vi "simularea_efectelor_grafice.vi"() -> ()   [LabVIEW 2025]
panel:
  out "DESCRIERE EFECT GRAFIC":string
  out "L 32":bool
  out "L 31":bool
  out "L 30":bool
  out "L 29":bool
  out "L 28":bool
  out "L 27":bool
  out "L 26":bool
  out "L 25":bool
  out "L 24":bool
  out "L 23":bool
  out "L 22":bool
  out "L 21":bool
  out "L 20":bool
  out "L 19":bool
  out "L 18":bool
  out "L 17":bool
  out "L 16":bool
  out "L 15":bool
  out "L 14":bool
  out "L 13":bool
  out "L 12":bool
  out "L 11":bool
  out "L 10":bool
  out "L 9":bool
  out "L 8":bool
  out "L 7":bool
  out "L 6":bool
  out "L 5":bool
  out "L 4":bool
  out "L 3":bool
  out "L 2":bool
  out "L 1":bool
  in  "VITEZA EFECT":i32(knob) scale=100.0..2000.0
  in  "SELECTOR-EFECTE GRAFICE":string(combo)
  in  "stop":bool
  # "marire dimensiune text -tastatura setata pe engleza(uk sau us)\n                                          - CTRL + SHIFT + >"
  # "SIMULAREA EFECTELOR GRAFICE CARE POT FI AFISATE LA NIVELUL MATRICEI CU 8x4 LEDURI"
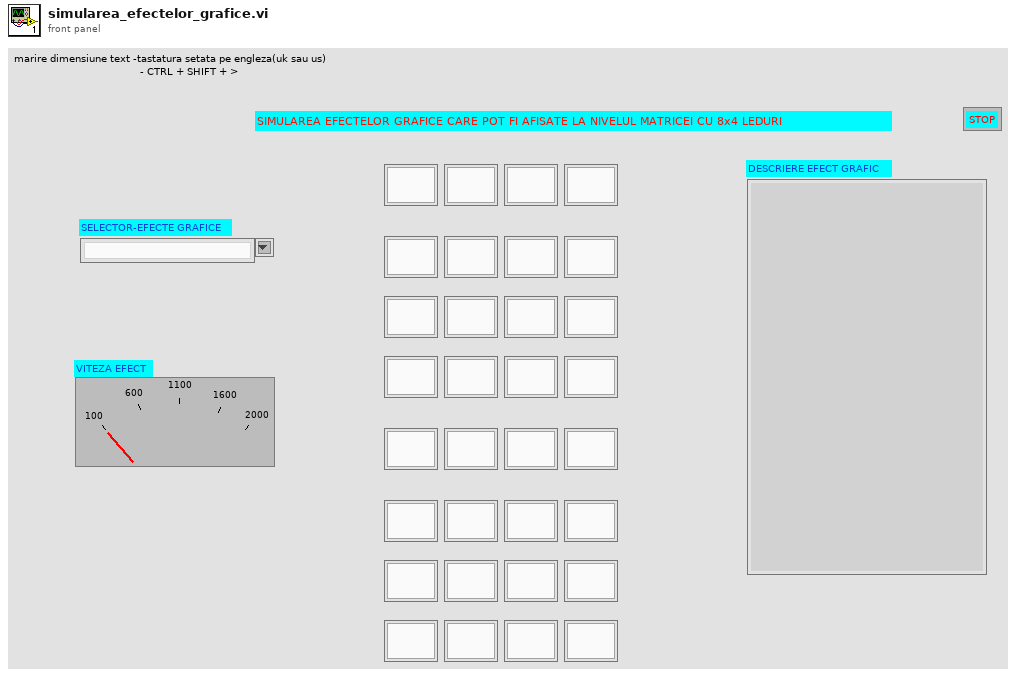
[diagram p1: front panel]
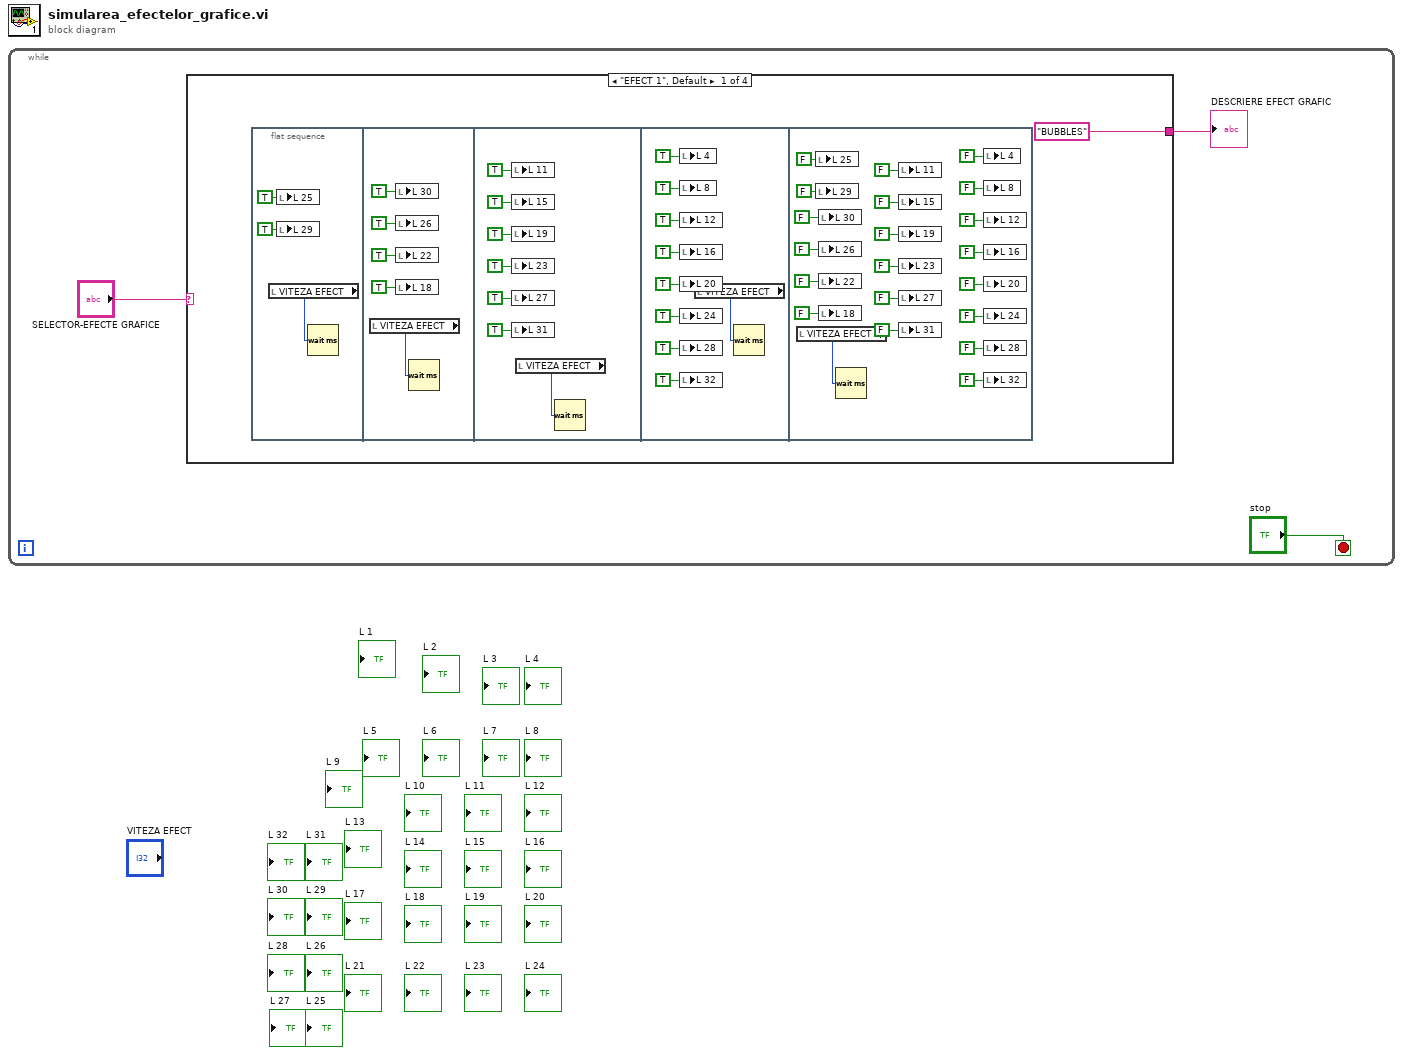
[diagram p0: block diagram]
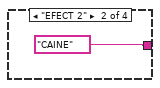
[diagram p2: hidden frame]
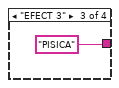
[diagram p3: hidden frame]
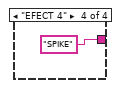
[diagram p4: hidden frame]
diagram:
  n1 = while {
    stop <- "stop" stop-if-true
    n2 = case shown="\"EFECT 1\", Default" "SELECTOR-EFECTE GRAFICE" {
      tunnel: ["BUBBLES" "CAINE" "PISICA" "SPIKE"] -> w1
      frame "EFECT 1", Default {
        n3 = flat-sequence {
          frame #0 {
            n4 = local read "VITEZA EFECT"() -> (w5:i32)
            n5 = local write "L 25"(TRUE ("L 25")) -> ()
            n6 = local write "L 29"(TRUE ("L 29")) -> ()
            n7 = Wait (ms)(milliseconds to wait=w5) -> ()  [unwired: 1 out]
          }
          frame #1 {
            n8 = local read "VITEZA EFECT"() -> (w8:i32)
            n9 = local write "L 30"(TRUE ("L 30")) -> ()
            n10 = local write "L 26"(TRUE ("L 26")) -> ()
            n11 = local write "L 22"(TRUE ("L 22")) -> ()
            n12 = local write "L 18"(TRUE ("L 18")) -> ()
            n13 = Wait (ms)(milliseconds to wait=w8) -> ()  [unwired: 1 out]
          }
          frame #2 {
            n14 = local write "L 11"(TRUE ("L 11")) -> ()
            n15 = local write "L 15"(TRUE ("L 15")) -> ()
            n16 = local write "L 19"(TRUE ("L 19")) -> ()
            n17 = local write "L 23"(TRUE ("L 23")) -> ()
            n18 = local write "L 27"(TRUE ("L 27")) -> ()
            n19 = local write "L 31"(TRUE ("L 31")) -> ()
            n20 = local read "VITEZA EFECT"() -> (w13:i32)
            n21 = Wait (ms)(milliseconds to wait=w13) -> ()  [unwired: 1 out]
          }
          frame #3 {
            n22 = local write "L 4"(TRUE ("L 4")) -> ()
            n23 = local write "L 8"(TRUE ("L 8")) -> ()
            n24 = local write "L 12"(TRUE ("L 12")) -> ()
            n25 = local write "L 16"(TRUE ("L 16")) -> ()
            n26 = local write "L 20"(TRUE ("L 20")) -> ()
            n27 = local write "L 24"(TRUE ("L 24")) -> ()
            n28 = local write "L 28"(TRUE ("L 28")) -> ()
            n29 = local write "L 32"(TRUE ("L 32")) -> ()
            n30 = local read "VITEZA EFECT"() -> (w20:i32)
            n31 = Wait (ms)(milliseconds to wait=w20) -> ()  [unwired: 1 out]
          }
          frame #4 {
            n32 = local read "VITEZA EFECT"() -> (w29:i32)
            n33 = local write "L 25"(FALSE ("L 25")) -> ()
            n34 = local write "L 29"(FALSE ("L 29")) -> ()
            n35 = local write "L 30"(FALSE ("L 30")) -> ()
            n36 = local write "L 26"(FALSE ("L 26")) -> ()
            n37 = local write "L 22"(FALSE ("L 22")) -> ()
            n38 = local write "L 18"(FALSE ("L 18")) -> ()
            n39 = Wait (ms)(milliseconds to wait=w29) -> ()  [unwired: 1 out]
            n40 = local write "L 11"(FALSE ("L 11")) -> ()
            n41 = local write "L 15"(FALSE ("L 15")) -> ()
            n42 = local write "L 19"(FALSE ("L 19")) -> ()
            n43 = local write "L 23"(FALSE ("L 23")) -> ()
            n44 = local write "L 27"(FALSE ("L 27")) -> ()
            n45 = local write "L 31"(FALSE ("L 31")) -> ()
            n46 = local write "L 4"(FALSE ("L 4")) -> ()
            n47 = local write "L 8"(FALSE ("L 8")) -> ()
            n48 = local write "L 12"(FALSE ("L 12")) -> ()
            n49 = local write "L 16"(FALSE ("L 16")) -> ()
            n50 = local write "L 20"(FALSE ("L 20")) -> ()
            n51 = local write "L 24"(FALSE ("L 24")) -> ()
            n52 = local write "L 28"(FALSE ("L 28")) -> ()
            n53 = local write "L 32"(FALSE ("L 32")) -> ()
          }
        }
      }
      frame "EFECT 2" {
      }
      frame "EFECT 3" {
      }
      frame "EFECT 4" {
      }
    }
    "DESCRIERE EFECT GRAFIC" <- w1
  }
